vi "DSF.Engine.Runtime.Framework.Initialize Cache.vi"(8 "error in (no error)":errorcluster, 11 "Framework Runtime in":refnum<class "DSF.Engine.Runtime.Framework.lvclass">) -> (0 "error out":errorcluster, 3 "Framework Runtime out":refnum<class "DSF.Engine.Runtime.Framework.lvclass">)   [LabVIEW 2016, in "DSF.Engine.lvlib" / "DSF.Engine.Runtime.Framework.lvclass"]
uses:
  DSF.Engine.Runtime.Framework.lvclass
  DSF.Engine.Runtime.Framework.lvclass/DSF.Engine.Runtime.Framework.ctl
  Cache/DSF.Engine.Memory.Cache.Framework.lvclass
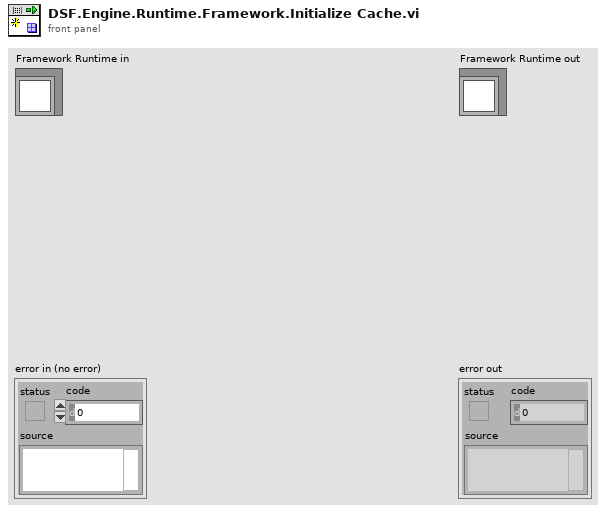
[diagram p1: front panel]
types:
  T1 = typedef "Custom Device API.lvlib/Custom Device Item Ref.ctl" = u64
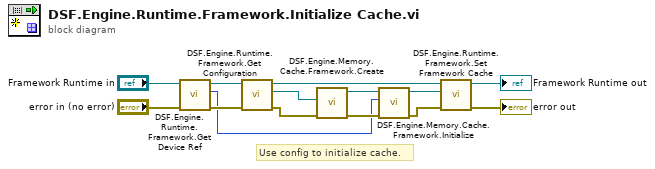
[diagram p0: block diagram]
diagram:
  # "Use config to initialize cache."
  n1 = call "DSF.Engine.Runtime.Framework.Get Device Ref.vi"("error in (no error)"="error in (no error)", "Framework Runtime in"="Framework Runtime in") -> ("error out"=w6:errorcluster, "Device Item Ref"=w1:T1, "Framework Runtime out"=w7:refnum<class "DSF.Engine.Runtime.Framework.lvclass">)  [unwired: 7 in]
  n2 = call "DSF.Engine.Runtime.Framework.Get Configuration.vi"("error in (no error)"=w6, "Framework Runtime in"=w7) -> ("error out"=w11:errorcluster, "Framework Configuration"=w12:refnum<class "DSF.Shared.Configuration.Framework.lvclass">, "Framework Runtime out"=w4:refnum<class "DSF.Engine.Runtime.Framework.lvclass">)  [unwired: 7 in]
  n3 = call "DSF.Engine.Memory.Cache.Framework.Create.vi"("error in (no error)"=w11, "Framework Configuration in"=w12) -> ("error out"=w5:errorcluster, "Framework Cache"=w10:refnum<class "DSF.Engine.Memory.Cache.Framework.lvclass">)  [unwired: 8 in]
  n4 = call "DSF.Engine.Memory.Cache.Framework.Initialize.vi"("error in (no error)"=w5, "Device Ref in"=w1, "Framework Cache in"=w10) -> ("error out"=w2:errorcluster, "Framework Cache out"=w3:refnum<class "DSF.Engine.Memory.Cache.Framework.lvclass">)  [unwired: 7 in]
  n5 = call "DSF.Engine.Runtime.Framework.Set Framework Cache.vi"("error in (no error)"=w2, "Framework Cache"=w3, "Framework Runtime in"=w4) -> ("error out"=→"error out":errorcluster, "Framework Runtime out"=→"Framework Runtime out":refnum<class "DSF.Engine.Runtime.Framework.lvclass">)  [unwired: 7 in]
